vi "TargetMatching(TargetsMingledotcom).vi"(10 "Left Targets":T1[](array[typedef]), 11 "Right Targets":T1[](array[typedef])) -> (3 "Target Set":T2(array[cluster]))   [LabVIEW 2014]
uses:
  target type.ctl
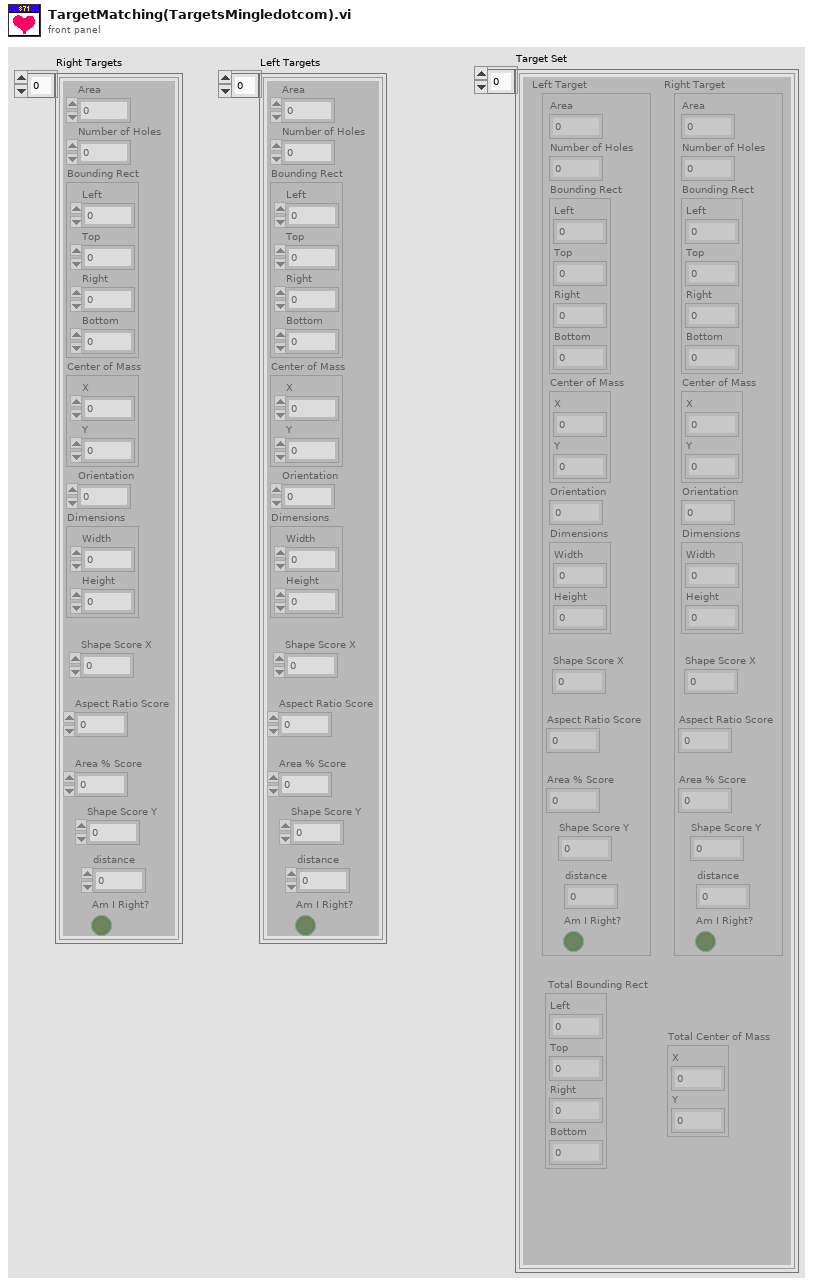
[diagram p1: front panel]
types:
  T1 = typedef "target type.ctl" = cluster{"Area":dbl, "Number of Holes":dbl, "Bounding Rect":cluster{"Left":dbl, "Top":dbl, "Right":dbl, "Bottom":dbl}, "Center of Mass":cluster{"X":dbl, "Y":dbl}, "Orientation":dbl, "Dimensions":cluster{"Width":dbl, "Height":dbl}, "Shape Score X":dbl, "Aspect Ratio Score":dbl, "Area % Score":dbl, "Shape Score Y":dbl, "Am I Right?":bool, "distance":dbl}
  T2 = cluster{"Left Target":T1, "Right Target":T1, "Total Bounding Rect":cluster{"Left":dbl, "Top":dbl, "Right":dbl, "Bottom":dbl}, "Total Center of Mass":cluster{"X":dbl, "Y":dbl}}[]
  T3 = cluster{"Left Target":T1, "Right Target":T1, "Total Bounding Rect":cluster{"Left":dbl, "Top":dbl, "Right":dbl, "Bottom":dbl}, "Total Center of Mass":cluster{"X":dbl, "Y":dbl}}
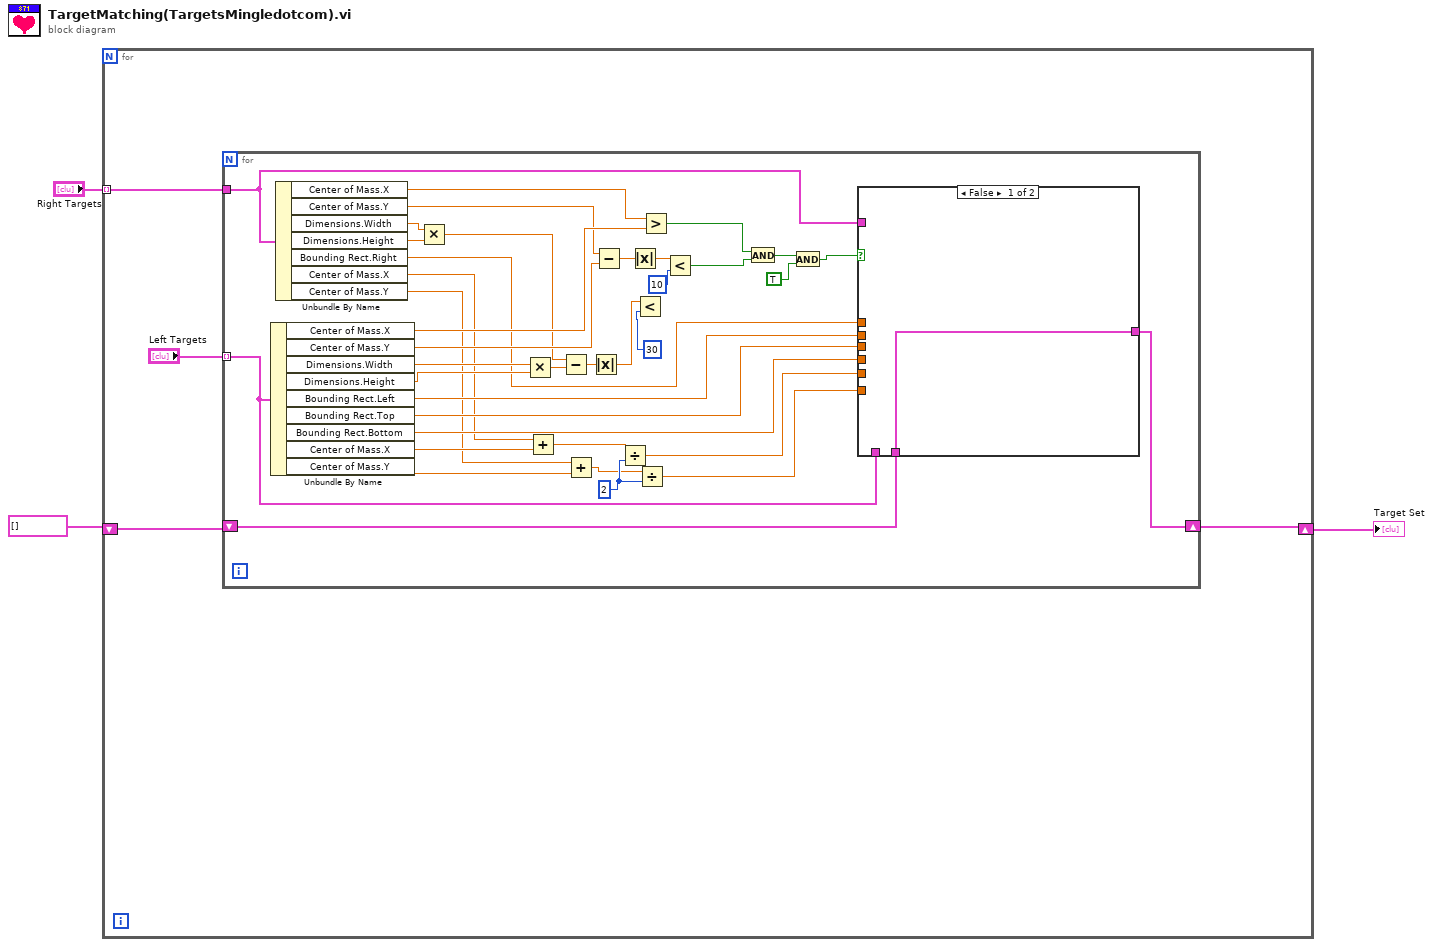
[diagram p0: block diagram]
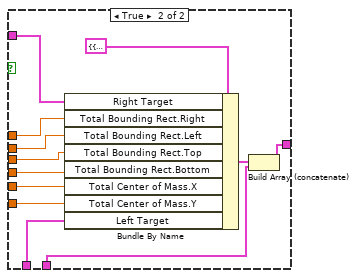
[diagram p2: hidden frame]
diagram:
  n1 = for {
    tunnel: "Right Targets" -> [w7] mode=indexing
    shift-right: [w4] -> w1
    shift-left: T2 [] -> [w5]
    n2 = for {
      tunnel: w7 -> [w29]
      tunnel: "Left Targets" -> [w28] mode=indexing
      shift-right: [w23] -> w4
      shift-left: w5 -> [w22]
      w16 = 2
      n3 = Unbundle By Name(w28) -> ("Center of Mass.X"=w44:dbl, "Center of Mass.Y"=w41:dbl, "Dimensions.Width"=w36:dbl, "Dimensions.Height"=w35:dbl, "Bounding Rect.Left"=w26:dbl, "Bounding Rect.Top"=w25:dbl, "Bounding Rect.Bottom"=w24:dbl, "Center of Mass.X"=w12:dbl, "Center of Mass.Y"=w11:dbl)
      n4 = Unbundle By Name(w29) -> ("Center of Mass.X"=w45:dbl, "Center of Mass.Y"=w42:dbl, "Dimensions.Width"=w38:dbl, "Dimensions.Height"=w37:dbl, "Bounding Rect.Right"=w27:dbl, "Center of Mass.X"=w13:dbl, "Center of Mass.Y"=w10:dbl)
      n5 = Multiply(x=w38, y=w37) -> (x*y=w33:dbl)
      n6 = Multiply(x=w36, y=w35) -> (x*y=w34:dbl)
      n7 = Add(x=w13, y=w12) -> (x+y=w14:dbl)
      n8 = Subtract(x=w33, y=w34) -> (x-y=w32:dbl)
      n9 = Add(x=w10, y=w11) -> (x+y=w15:dbl)
      n10 = Absolute Value(x=w32) -> (abs(x)=w21:dbl)
      n11 = Subtract(x=w42, y=w41) -> (x-y=w43:dbl)
      n12 = Divide(x=w14, y=w16) -> (x/y=w9:dbl)
      n13 = Absolute Value(x=w43) -> (abs(x)=w19:dbl)
      n14 = Less?(x=w21, y=30) -> ()  [unwired: 1 out]
      n15 = Divide(x=w15, y=w16) -> (x/y=w8:dbl)
      n16 = Greater?(x=w45, y=w44) -> (0:w40:bool)
      n17 = Less?(x=w19, y=10) -> (x < y?=w39:bool)
      n18 = And(x=w40, y=w39) -> (x .and. y?=w31:bool)
      n19 = And(x=w31, y=TRUE) -> (x .and. y?=w30:bool)
      n20 = case shown="False" w30 {
        tunnel: w29 -> [_ w54]
        tunnel: w28 -> [_ w52]
        tunnel: [w46 w49] -> w23
        tunnel: w27 -> [_ w58]
        tunnel: w26 -> [_ w57]
        tunnel: w25 -> [_ w56]
        tunnel: w24 -> [_ w55]
        tunnel: w22 -> [w46 w47]
        tunnel: w9 -> [_ w51]
        tunnel: w8 -> [_ w50]
        frame False {
        }
        frame True {
          n21 = Bundle By Name(cluster=T3 {"Left Target"={"Area"=0.0, "Number of Holes"=0.0, "Bounding Rect"={"Left"=0.0, "Top"=0.0, "Right"=0.0, "Bottom"=0.0}, "Center of Mass"={"X"=0.0, "Y"=0.0}, "Orientation"=0.0, "Dimensions"={"Width"=0.0, "Height"=0.0}, "Shape Score X"=0.0, "Aspect Ratio Score"=0.0, "Area % Score"=0.0, "Shape Score Y"=0.0, "Am I Right?"=FALSE, "distance"=0.0}, "Right Target"={"Area"=0.0, "Number of Holes"=0.0, "Bounding Rect"={"Left"=0.0, "Top"=0.0, "Right"=0.0, "Bottom"=0.0}, "Center of Mass"={"X"=0.0, "Y"=0.0}, "Orientation"=0.0, "Dimensions"={"Width"=0.0, "Height"=0.0}, "Shape Score X"=0.0, "Aspect Ratio Score"=0.0, "Area % Score"=0.0, "Shape Score Y"=0.0, "Am I Right?"=FALSE, "distance"=0.0}, "Total Bounding Rect"={"Left"=0.0, "Top"=0.0, "Right"=0.0, "Bottom"=0.0}, "Total Center of Mass"={"X"=0.0, "Y"=0.0}} ("Cluster"), "Right Target"=w54, "Total Bounding Rect.Right"=w58, "Total Bounding Rect.Left"=w57, "Total Bounding Rect.Top"=w56, "Total Bounding Rect.Bottom"=w55, "Total Center of Mass.X"=w51, "Total Center of Mass.Y"=w50, "Left Target"=w52) -> (w48:T3)
          n22 = Build Array (concatenate)(w48, w47) -> (w49:T2)
        }
      }
    }
  }
  "Target Set" <- w1
